vi "Digital Output 7 Segment.vi"() -> ()   [LabVIEW 2012]
uses:
  <vilib>/DAQmx/write.llb/DAQmx Write (Digital 1D Bool NChan 1Samp 1Line).vi
  <vilib>/DAQmx/create/channels.llb/DAQmx Create Channel (DO-Digital Output).vi
  <vilib>/DAQmx/miscellaneous.llb/DAQmx Fill In Error Info.vi
panel:
  in  "?":bool
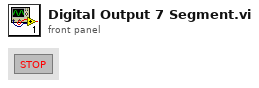
[diagram p1: front panel]
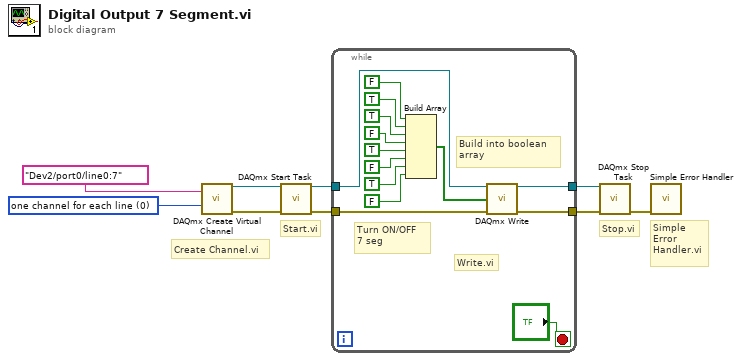
[diagram p0: block diagram]
diagram:
  w9 = 0 items=["one channel for each line", "one channel for all lines"] ("line grouping")
  # "Simple\nError\nHandler.vi"
  # "Stop.vi"
  # "Start.vi"
  # "Create Channel.vi"
  n1 = call-poly <vilib>:"DAQmx Create Virtual Channel.vi"("lines"=tag "Dev2/port0/line0:7", "line grouping"=w9) -> ("task out"=w8:refnum<k21>, "error out"=w7:errorcluster)  [unwired: 12 in]
  n2 = call <vilib>:"DAQmx Start Task.vi"("task/channels in"=w8, "error in"=w7) -> ("task out"=w6:refnum<k21>, "error out"=w5:errorcluster)  [unwired: 12 in]
  n3 = while {
    tunnel: w6 -> [w20]
    tunnel: w5 -> [w10]
    tunnel: [w23] -> w4
    tunnel: [w22] -> w3
    stop <- "?" stop-if-true
    # "Turn ON/OFF\n7 seg"
    # "Build into boolean array"
    # "Write.vi"
    n4 = Build Array(FALSE, TRUE, TRUE, FALSE, TRUE, FALSE, TRUE, FALSE) -> (w11:bool[])
    n5 = call-poly <vilib>:"DAQmx Write.vi"("task/channels in"=w20, "data"=w11, "error in"=w10) -> ("task out"=w23:refnum<k21>, "error out"=w22:errorcluster)  [unwired: 10 in, 1 out]
  }
  n6 = call <vilib>:"DAQmx Stop Task.vi"("task/channels in"=w4, "error in"=w3) -> ("error out"=w2:errorcluster)  [unwired: 12 in, 1 out]
  n7 = call <vilib>:"Simple Error Handler.vi"("error in (no error)"=w2) -> ()  [unwired: 4 in, 5 out]
